vi "Empty Array.vi"(7 "Dispose Elements? (T)":bool=TRUE, 8 "error in (no error)":errorcluster, 11 "ArrayManager in":refnum<class "ArrayManager.lvclass">) -> (0 "error out":errorcluster, 3 "ArrayManager out":refnum<class "ArrayManager.lvclass">)   [LabVIEW 2020, in "OOPanel.lvlib" / "ArrayManager.lvclass"]
uses:
  ArrayManager.lvclass
  ArrayManager.lvclass/ArrayManager.ctl
  ArrayPanel/ArrayPanel.lvclass
  Manager/Manager.lvclass
  C:/dev/IlluminatedG/.lv-oopanel/OOPanel/Panel/Panel.lvclass
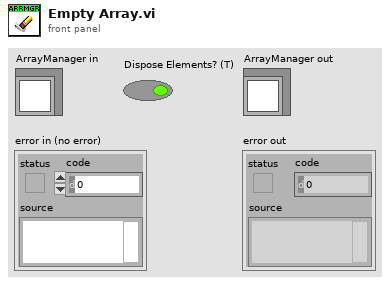
[diagram p1: front panel]
types:
  T1 = typedef "OOPanel.lvlib/ArrayManager.lvclass/State Ref.ctl" = cluster{"Running":bool, "Borders":bool, "Total Height":dbl, "Scroll Visible":bool, "Background":u32}
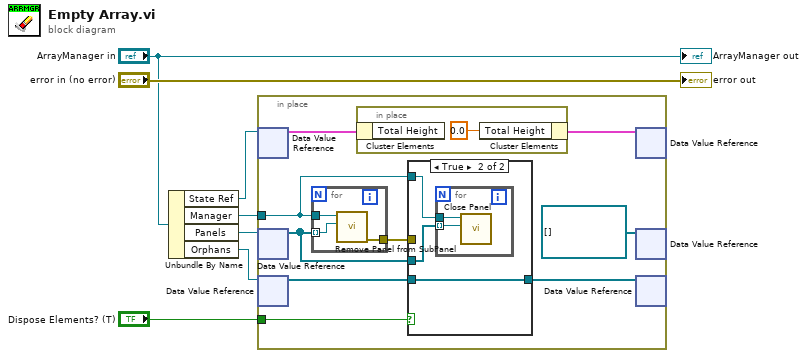
[diagram p0: block diagram]
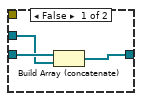
[diagram p2: hidden frame]
diagram:
  n1 = Unbundle By Name("ArrayManager in") -> ("State Ref"=w1:refnum<data-value>, "Manager"=w4:refnum<class "Manager.lvclass">, "Panels"=w6:refnum<data-value>, "Orphans"=w3:refnum<data-value>)
  n2 = in-place {
    in-place-border: w4 -> [w12]
    in-place-border: "Dispose Elements? (T)" -> [w14]
    n3 = in-place-dvr #1(w1) -> (w10:T1)  [unwired: 1 out]
    n4 = in-place-dvr #2(w6) -> (w13:refnum<class "ArrayPanel.lvclass">[])  [unwired: 1 out]
    n5 = in-place-dvr #3(w3) -> (w15:refnum<class "ArrayPanel.lvclass">[])  [unwired: 1 out]
    n6 = for {
      tunnel: w12 -> [w28]
      tunnel: w13 -> [w27] mode=indexing
      tunnel: [w26] -> w8
      n7 = call "Remove Panel from SubPanel.vi"("Panel In"=w27, "Manager in"=w28) -> ("error out"=w26:errorcluster)  [unwired: 7 in, 2 out]
    }
    n8 = in-place {
      n9 = in-place-cluster #4(w10) -> ()  [unwired: 1 out]
      n10 = in-place-cluster #4("Total Height"=0.0) -> (w9:T1)
    }
    n11 = case shown="True" w14 {
      tunnel: w15 -> [w20 w23]
      tunnel: w13 -> [w19 w21]
      tunnel: w12 -> [_ w22]
      tunnel: [w18 w23] -> w11
      tunnel: w8 -> [_ _]
      frame False {
        n12 = Build Array (concatenate)(w20, w19) -> (w18:refnum<class "ArrayPanel.lvclass">[])
      }
      frame True {
        n13 = for {
          tunnel: w22 -> [w25]
          tunnel: w21 -> [w24] mode=indexing
          n14 = call "Close Panel.vi"("Panel"=w24, "Manager in"=w25) -> ()  [unwired: 8 in, 2 out]
        }
      }
    }
    n15 = in-place-dvr #1(w9) -> ()  [unwired: 2 out]
    n16 = in-place-dvr #2(refnum<class "ArrayPanel.lvclass">[] [] ("data value")) -> ()  [unwired: 2 out]
    n17 = in-place-dvr #3(w11) -> ()  [unwired: 2 out]
  }
  "error out" <- "error in (no error)"
  "ArrayManager out" <- "ArrayManager in"
